vi "Thresholding.vi"(8 "error in (no error)":errorcluster, 10 "Threshold Value":sgl=1.0 format="%.2f", 11 "Image Src":T1) -> (0 "error out":errorcluster, 3 "Image":T1(plugin-control))   [LabVIEW 2017]
uses:
  <vilib>/vision/Image Controls.llb/IMAQ Image.ctl
  <vilib>/vision/NI_Vision_Development_Module.lvlib
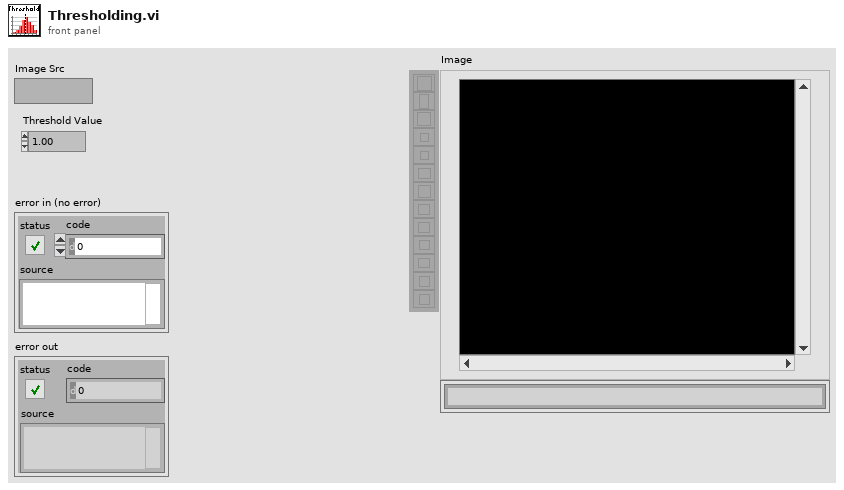
[diagram p1: front panel]
types:
  T1 = typedef "IMAQ Image.ctl" = refnum<image>
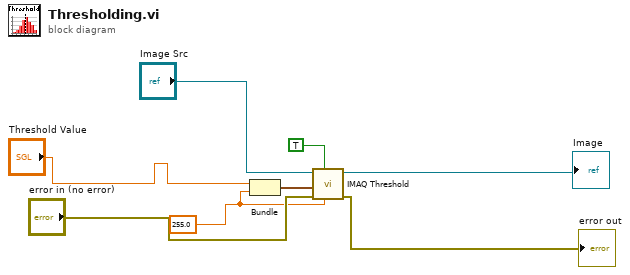
[diagram p0: block diagram]
diagram:
  w3 = sgl 255.0
  n1 = Bundle("Threshold Value"="Threshold Value", w3) -> (w6:cluster{"Threshold Value":sgl, sgl})  [unwired: 1 in]
  n2 = call "IMAQ Threshold"("Replace Value"=w3, "Keep/Replace Value (Replace)"=TRUE, "error in (no error)"="error in (no error)", "Range"=w6, "Image Src"="Image Src") -> ("error out"=→"error out":errorcluster, "Image Dst Out"=→"Image":T1)  [unwired: 5 in]
